vi "WriteInputTunnels.vi"(5 "inputs":refnum<class "Tunnel.lvclass">[](array[class]), 9 "Structure in":refnum<class "Structure.lvclass">) -> (3 "Structure out":refnum<class "Structure.lvclass">)   [LabVIEW 2014, in "Structure.lvclass"]
uses:
  Structure.lvclass
  Tunnel/Tunnel.lvclass
  Structure.lvclass/Structure.ctl
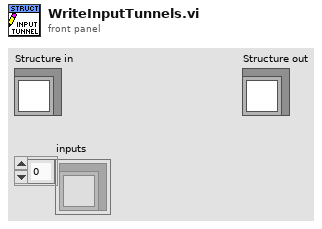
[diagram p1: front panel]
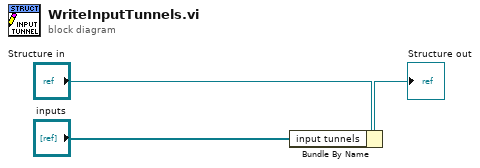
[diagram p0: block diagram]
diagram:
  n1 = Bundle By Name(cluster="Structure in", "input tunnels"="inputs") -> (→"Structure out":refnum<class "Structure.lvclass">)
